vi "flash_lamp (SubVI).vi"(8 "Flash lamp\n settings:":T1={"Flash lamp?"=FALSE, "Number of cyles\nbetween flashes"=3, "# Pulses"=35, "Stop flashing \nbelow thresh?"=FALSE, "Stop threshold"=0.001, "Pulse voltage?"=FALSE, "Pulse length (ms)"=0.001, "Pulse amp (V)"=0.001}, 9 "# Pulses in":i32, 11 "Output channel (for flashing)":tag) -> ()   [LabVIEW 2014]
uses:
  <vilib>/DAQmx/create/channels.llb/DAQmx Create Channel (AO-Voltage-Basic).vi
  <vilib>/DAQmx/configure/timing.llb/DAQmx Timing (Sample Clock).vi
  <vilib>/DAQmx/write.llb/DAQmx Write (Analog 2D DBL NChan NSamp).vi
  <vilib>/DAQmx/write.llb/DAQmx Write (Analog 1D DBL 1Chan NSamp).vi
panel:
  out "Waveform Graph":dbl[](graph)
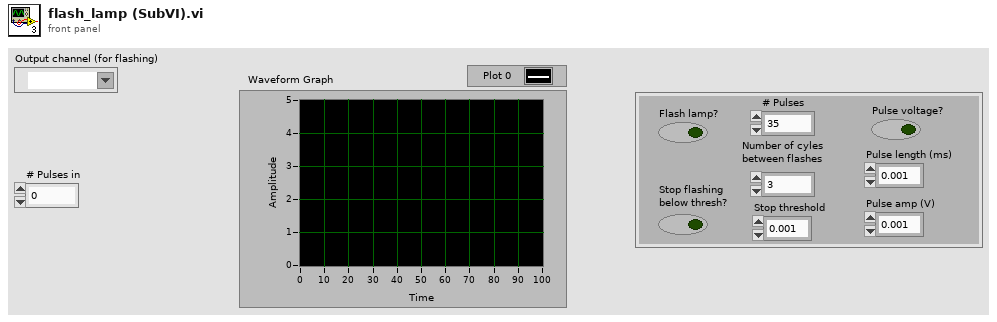
[diagram p1: front panel]
types:
  T1 = cluster{"Flash lamp?":bool, "Number of cyles\nbetween flashes":i32, "# Pulses":i32, "Stop flashing \nbelow thresh?":bool, "Stop threshold":dbl, "Pulse voltage?":bool, "Pulse length (ms)":dbl, "Pulse amp (V)":dbl}
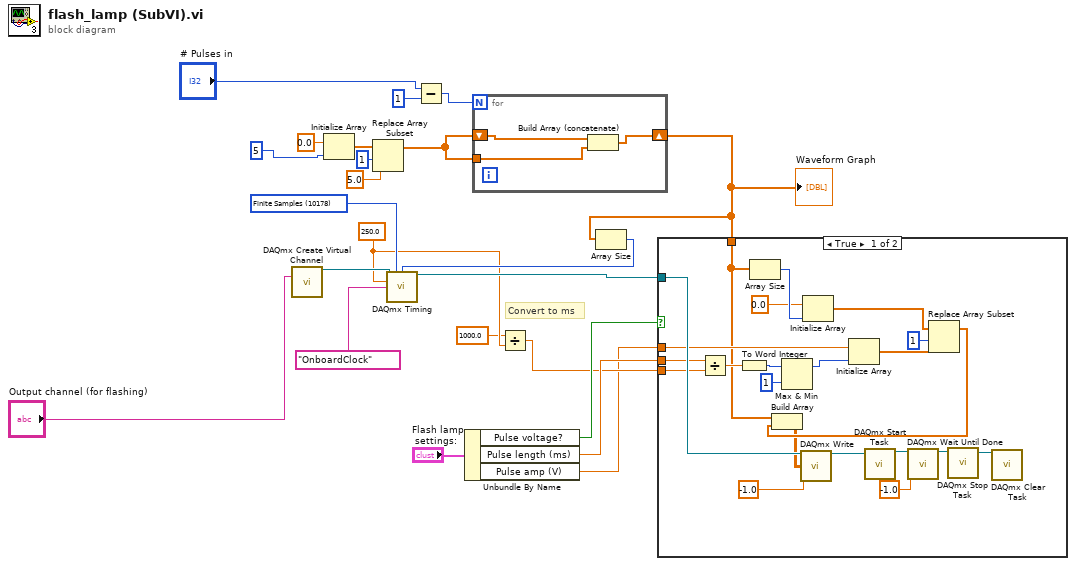
[diagram p0: block diagram]
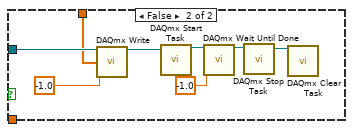
[diagram p2: hidden frame]
diagram:
  w13 = 10178 items=["Finite Samples"=10178, "Continuous Samples"=10123, "Hardware Timed Single Point"=12522] ("sample mode")
  w5 = 250.0 ("Sample Rate")
  # "Convert to ms"
  n1 = call-poly <vilib>:"DAQmx Create Virtual Channel.vi"("physical channels"="Output channel (for flashing)") -> ("task out"=w22:refnum<k21>)  [unwired: 13 in, 1 out]
  n2 = Initialize Array(0.0 ("element"), 5 ("y")) -> (w18:dbl[])
  n3 = Replace Array Subset(array=w18, new element=5.0 ("new element/subarray"), index=1) -> (w15:dbl[])
  n4 = Subtract(x="# Pulses in", y=1) -> (x-y=w10:i32)
  n5 = Unbundle By Name("Flash lamp\n settings:") -> ("Pulse voltage?"=w7:bool, "Pulse length (ms)"=w6:dbl, "Pulse amp (V)"=w1:dbl)
  n6 = for {
    N: w10 -> [_]
    shift-right: [w24] -> w2
    shift-left: w15 -> [w26]
    tunnel: w15 -> [w25]
    n7 = Build Array (concatenate)(w26, w25) -> (w24:dbl[])
  }
  "Waveform Graph" <- w2
  n8 = Divide(x=1000.0, y=w5) -> (x/y=w3:dbl)
  n9 = Array Size(array=w2) -> (size(s)=w12:i32)
  n10 = call-poly <vilib>:"DAQmx Timing.vi"("task/channels in"=w22, "sample mode"=w13, "samples per channel"=w12, "rate"=w5, "source"=tag "OnboardClock") -> ("task out"=w20:refnum<k21>)  [unwired: 9 in, 1 out]
  n11 = case shown="True" w7 {
    tunnel: w20 -> [w42 w50]
    tunnel: w2 -> [w29 w49]
    tunnel: w1 -> [w39 _]
    tunnel: w6 -> [w38 _]
    tunnel: w3 -> [w37 _]
    frame True {
      n12 = Divide(x=w38, y=w37) -> (x/y=w36:dbl)
      n13 = To Word Integer(number=w36) -> (16bit integer=w35:i16)
      n14 = Array Size(array=w29) -> (size(s)=w41:i32)
      n15 = Max & Min(x=w35, y=i16 1) -> (max(x,y)=w33:i16)  [unwired: 1 out]
      n16 = Initialize Array(0.0 ("element"), w41) -> (w30:dbl[])
      n17 = Initialize Array(w39, w33) -> (w32:dbl[])
      n18 = Replace Array Subset(array=w30, new element=w32, index=1) -> (w28:dbl[])
      n19 = Build Array(w29, w28) -> (w27:dbl[][])
      n20 = call-poly <vilib>:"DAQmx Write.vi"("task/channels in"=w42, "data"=w27, "timeout"=-1.0) -> ("task out"=w47:refnum<k21>)  [unwired: 10 in, 2 out]
      n21 = call <vilib>:"DAQmx Start Task.vi"("task/channels in"=w47) -> ("task out"=w46:refnum<k21>)  [unwired: 13 in, 1 out]
      n22 = call <vilib>:"DAQmx Wait Until Done.vi"("task/channels in"=w46, "timeout (sec)"=-1.0) -> ("task out"=w45:refnum<k21>)  [unwired: 12 in, 1 out]
      n23 = call <vilib>:"DAQmx Stop Task.vi"("task/channels in"=w45) -> ("task out"=w48:refnum<k21>)  [unwired: 13 in, 1 out]
      n24 = call <vilib>:"DAQmx Clear Task.vi"("task in"=w48) -> ()  [unwired: 14 in, 1 out]
    }
    frame False {
      n25 = call-poly <vilib>:"DAQmx Write.vi"("task/channels in"=w50, "data"=w49, "timeout"=-1.0) -> ("task out"=w55:refnum<k21>)  [unwired: 10 in, 2 out]
      n26 = call <vilib>:"DAQmx Start Task.vi"("task/channels in"=w55) -> ("task out"=w54:refnum<k21>)  [unwired: 13 in, 1 out]
      n27 = call <vilib>:"DAQmx Wait Until Done.vi"("task/channels in"=w54, "timeout (sec)"=-1.0) -> ("task out"=w53:refnum<k21>)  [unwired: 12 in, 1 out]
      n28 = call <vilib>:"DAQmx Stop Task.vi"("task/channels in"=w53) -> ("task out"=w56:refnum<k21>)  [unwired: 13 in, 1 out]
      n29 = call <vilib>:"DAQmx Clear Task.vi"("task in"=w56) -> ()  [unwired: 14 in, 1 out]
    }
  }
